vi "Num Ref Update Color.vi"(8 "error in (no error)":errorcluster, 11 "Num ref":refnum<vi>) -> (0 "error out":errorcluster)   [LabVIEW 2018, in "LF2R IDE.lvlib" / "LF2R IDE.lvclass"]
uses:
  LF2R IDE.lvclass
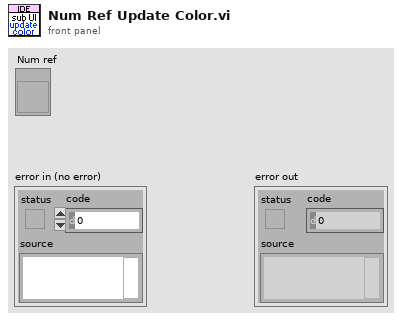
[diagram p1: front panel]
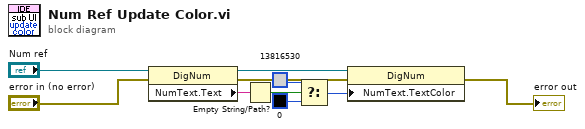
[diagram p0: block diagram]
diagram:
  n1 = property class="DigNum"(reference="Num ref", error in="error in (no error)") -> (reference out=w7:refnum<vi>, error out=w1:errorcluster, "NumText.Text"=w6:string)
  n2 = Empty String/Path?(string/path=w6) -> (empty?=w5:bool)
  n3 = Select(t=u32 13816530, s=w5, f=u32 0) -> (s? t:f=w2:u32)
  n4 = property class="DigNum"(reference=w7, error in=w1, "NumText.TextColor"=w2) -> (error out=→"error out":errorcluster)  [unwired: 1 out]
